vi "Tester.vi"() -> ()   [LabVIEW 2016]
uses:
  <vilib>/FPGAPlugInAG/cRIO-9039 (Sync)/niLvFpga_Open_cRIO-9039 (Sync).vi
  <vilib>/rvi/interface/common/dynamic/niFpgaDynamicAddResources.vi
  <vilib>/Utility/error.llb/Error Cluster From Error Code.vi
  <vilib>/rvi/errors/niLvFpgaAdjustHostInterfaceError.vi
  <vilib>/rvi/interface/nirviOpenFPGA/nirviOpenFPGA.xnode
  FPGA Bitfiles/IntelliRupter_calibrated.lvbitx
  <vilib>/rvi/interface/nirviReadWriteControl/nirviReadWriteControl.xnode
  <vilib>/rvi/interface/Simulation/niFpgaSimulationCallBeginRW.vi
  NiFpgaLv.dll
panel:
  out "Waveform Chart 2":dynamicdata(graph)
  out "Active Power":dbl
  out "x-y":u32=48
  out "RMS":fxp<+,55,5>
  out "frequency":dbl
  in  "fc":dbl
  out "Waveform Chart":dynamicdata(graph)
  in  "stop":bool
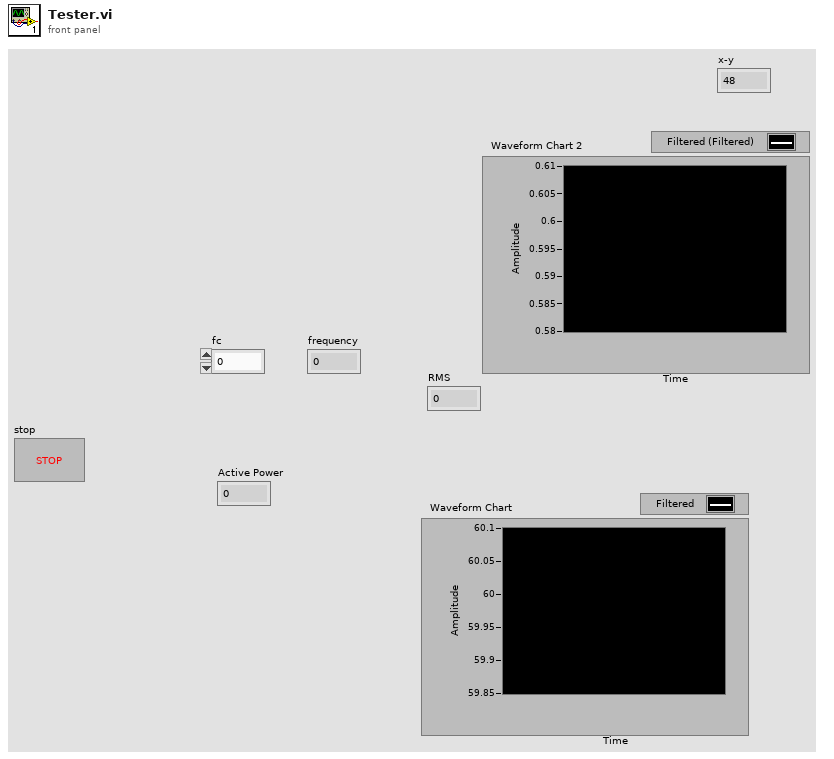
[diagram p1: front panel]
types:
  T1 = cluster{"V1L AB":fxp<+/-,53,11>, "V1L BC":fxp<+/-,53,11>, "V1L CA":fxp<+/-,53,11>}
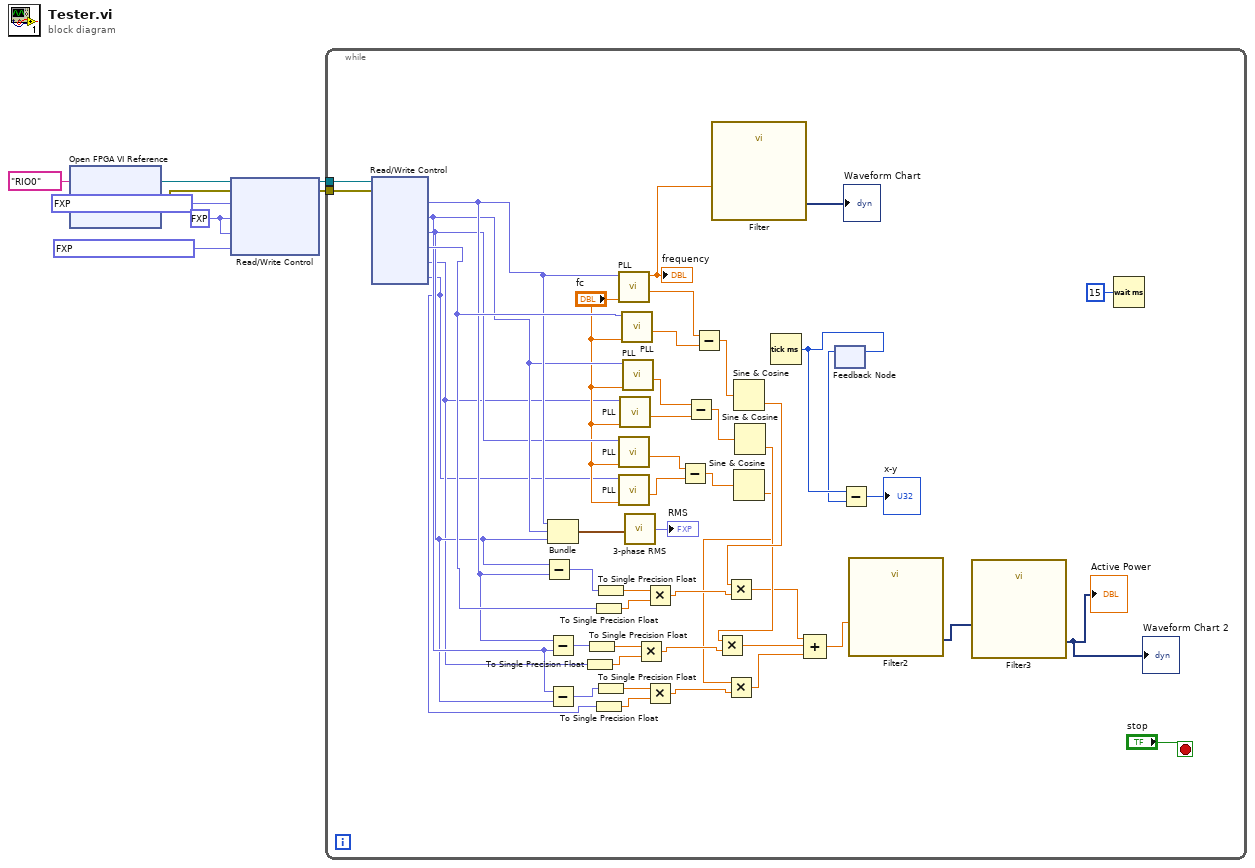
[diagram p0: block diagram]
diagram:
  w3 = fxp<+/-,52,10> 0.0 ("I offset")
  n1 = xnode "Open FPGA VI Reference"("resource name"=tag "RIO0") -> ("FPGA VI Reference Out"=w8:refnum<k20>, "error out"=w6:errorcluster)  [unwired: 1 in]
  n2 = xnode "Read/Write Control"("FPGA VI Reference In"=w8, "error in"=w6, "I scale factor"=fxp<+/-,26,5> 0.4850001335144043, "I offset"=w3, "V offset"=w3, "V scale factor"=fxp<+/-,26,5> 0.40000009536743164) -> ("FPGA VI Reference Out"=w2:refnum<k20>, "error out"=w1:errorcluster)
  n3 = while {
    tunnel: w2 -> [w55]
    tunnel: w1 -> [w54]
    stop <- "stop" stop-if-true
    n4 = xnode "Read/Write Control"("FPGA VI Reference In"=w55, "error in"=w54) -> ("V1L AB"=w37:fxp<+/-,53,11>, "V1L BC"=w36:fxp<+/-,53,11>, "V1L CA"=w35:fxp<+/-,53,11>, "I1 A"=w43:fxp<+/-,53,11>, "I1 B"=w20:fxp<+/-,53,11>, "I1 C"=w18:fxp<+/-,53,11>)  [unwired: 2 out]
    n5 = Subtract(x=w35, y=w37) -> (x-y=w46:fxp<+/-,53,11>)
    n6 = Bundle("V1L AB"=w37, "V1L BC"=w36, "V1L CA"=w35) -> (w51:T1)  [unwired: 1 in]
    n7 = Subtract(x=w37, y=w36) -> (x-y=w21:fxp<+/-,53,11>)
    n8 = Subtract(x=w36, y=w35) -> (x-y=w19:fxp<+/-,53,11>)
    n9 = To Single Precision Float(number=w20) -> (single precision float=w26:sgl)
    n10 = To Single Precision Float(number=w21) -> (single precision float=w25:sgl)
    n11 = To Single Precision Float(number=w43) -> (single precision float=w44:sgl)
    n12 = To Single Precision Float(number=w18) -> (single precision float=w23:sgl)
    n13 = To Single Precision Float(number=w46) -> (single precision float=w45:sgl)
    n14 = To Single Precision Float(number=w19) -> (single precision float=w24:sgl)
    n15 = call "PLL.vi"("fc"="fc", "input"=w37) -> ("phase"=w42:dbl, "frequency"=w53:dbl)  [unwired: 8 in]
    "frequency" <- w53
    n16 = call "PLL.vi"("fc"="fc", "input"=w35) -> ("phase"=w33:dbl)  [unwired: 8 in, 1 out]
    n17 = call "PLL.vi"("fc"="fc", "input"=w18) -> ("phase"=w32:dbl)  [unwired: 8 in, 1 out]
    n18 = call "PLL.vi"("fc"="fc", "input"=w20) -> ("phase"=w30:dbl)  [unwired: 8 in, 1 out]
    n19 = call "PLL.vi"("fc"="fc", "input"=w43) -> ("phase"=w41:dbl)  [unwired: 8 in, 1 out]
    n20 = call "PLL.vi"("fc"="fc", "input"=w36) -> ("phase"=w31:dbl)  [unwired: 8 in, 1 out]
    n21 = call "3-phase RMS.vi"("Vabc"=w51) -> ("RMS"=→"RMS":fxp<+,55,5>)  [unwired: 4 in]
    n22 = Multiply(x=w25, y=w26) -> (x*y=w27:sgl)
    n23 = Multiply(x=w45, y=w44) -> (x*y=w39:sgl)
    n24 = Multiply(x=w24, y=w23) -> (x*y=w22:sgl)
    n25 = Subtract(x=w33, y=w32) -> (x-y=w28:dbl)
    n26 = Subtract(x=w31, y=w30) -> (x-y=w29:dbl)
    n27 = Subtract(x=w42, y=w41) -> (x-y=w40:dbl)
    n28 = call "Filter"("Signal"=w53) -> ("Filtered Signal"=→"Waveform Chart":dynamicdata)  [unwired: 9 in, 1 out]
    n29 = Sine & Cosine(0:w40) -> (2:w38:dbl)  [unwired: 1 out]
    n30 = Multiply(x=w38, y=w39) -> (x*y=w13:dbl)
    n31 = Sine & Cosine(0:w28) -> (2:w16:dbl)  [unwired: 1 out]
    n32 = Multiply(x=w16, y=w22) -> (x*y=w15:dbl)
    n33 = Sine & Cosine(0:w29) -> (2:w17:dbl)  [unwired: 1 out]
    n34 = Multiply(x=w17, y=w27) -> (x*y=w14:dbl)
    n35 = Tick Count (ms)() -> (millisecond timer value=w48:u32)
    n36 = Compound Arithmetic op=ADD(w13, w14, w15) -> (w12:dbl)
    n37 = feedback #1() -> (w47:u32)  [unwired: 1 in]
    n38 = feedback-in #1(w48) -> ()
    n39 = Subtract(x=w48, y=w47) -> (x-y=→"x-y":u32)
    n40 = call "Filter2"("Signal"=w12) -> ("Filtered Signal"=w11:dynamicdata)  [unwired: 9 in, 1 out]
    n41 = call "Filter3"("Signal"=w11) -> ("Filtered Signal"=→"Active Power" →"Waveform Chart 2":dynamicdata)  [unwired: 9 in, 1 out]
    n42 = Wait (ms)(milliseconds to wait=u32 15) -> ()  [unwired: 1 out]
  }
